vi "GetNamedNumericReference.vi"(8 "error in":errorcluster, 11 "NamedNumeric in":refnum<class "NamedNumeric.lvclass">) -> (0 "error out":errorcluster, 1 "Named Numeric reference":refnum<vi>, 3 "NamedNumeric out":refnum<class "NamedNumeric.lvclass">)   [LabVIEW 2014, in "Raspberry Pi Compatible Compiler for LabVIEW.lvlib" / "NamedNumeric.lvclass"]
uses:
  NamedNumeric.lvclass
  Generic/Generic.lvclass
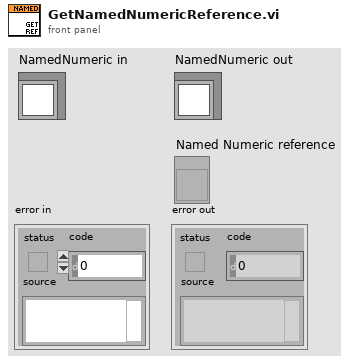
[diagram p1: front panel]
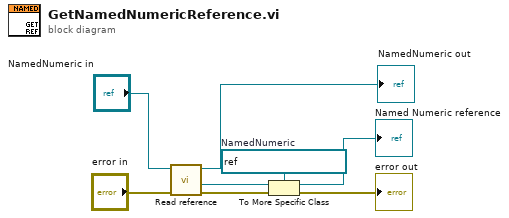
[diagram p0: block diagram]
diagram:
  w8 = refnum<vi> refnum  # NamedNumeric
  n1 = call "Read reference.vi"("error in"="error in", "GObject in"="NamedNumeric in") -> ("error out"=w3:errorcluster, "reference"=w2:refnum<vi>, "GObject out"=→"NamedNumeric out":refnum<class "NamedNumeric.lvclass">)  [unwired: 5 in]
  n2 = To More Specific Class(target class=w8, reference=w2, error in=w3) -> (specific class reference=→"Named Numeric reference":refnum<vi>, error out=→"error out":errorcluster)
